vi "UI_spinWheel.vi"(8 "error in (no error)":errorcluster) -> (0 "error out":errorcluster, 2 "Cash":dbl, 3 "Spin Result":string)   [LabVIEW 2020]
uses:
  Typedefs/game_wheelItems.ctl
  <vilib>/numeric/Random Number (Range) U64.vi
  <vilib>/numeric/sub_Random U32.vi
panel:
  in  "OK":bool
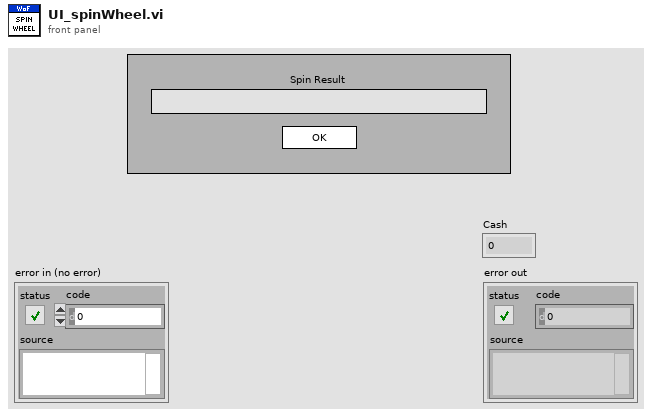
[diagram p1: front panel]
types:
  T1 = typedef "game_wheelItems.ctl" = string[]
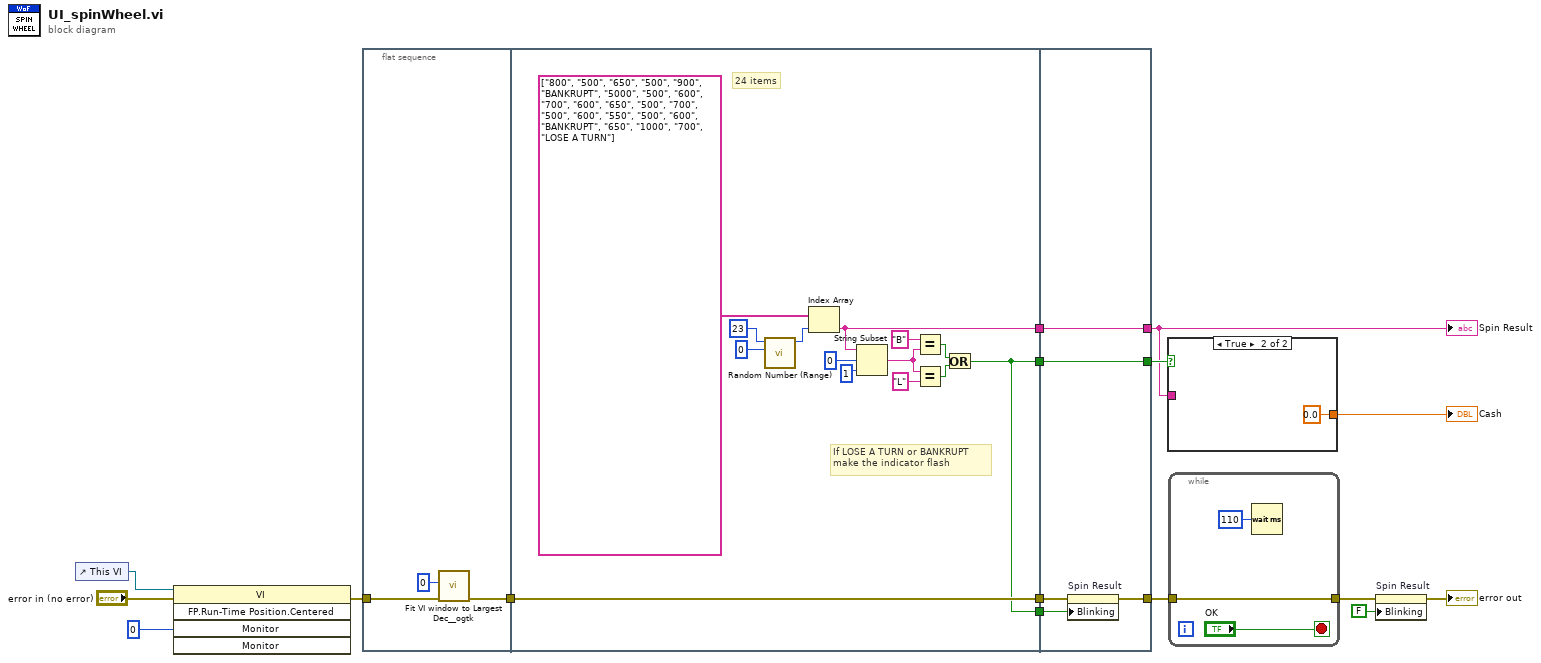
[diagram p0: block diagram]
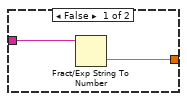
[diagram p2: hidden frame]
diagram:
  n1 = control-ref of="This VI"() -> (w1:refnum<vi>)
  n2 = invoke class="VI" method="FP.Run-Time Position.Centered"(reference=w1, error in="error in (no error)", "Monitor"=i16 0) -> (error out=w4:errorcluster)  [unwired: 2 in, 4 out]
  n3 = flat-sequence {
    tunnel: w4 -> [w18]
    tunnel: [w17] -> w16
    tunnel: w16 -> [w29]
    tunnel: [w29] -> w15
    tunnel: [w28] -> w13
    tunnel: [w20] -> w9
    tunnel: [w20] -> w8
    tunnel: w15 -> [w37]
    tunnel: [w36] -> w14
    tunnel: w13 -> [w38]
    tunnel: [w38] -> w6
    tunnel: w9 -> [w35]
    tunnel: w8 -> [w34]
    tunnel: [w34] -> w7
    frame #0 {
      n4 = call <userlib>:"Fit VI window to Largest Dec__ogtk.vi"("error in (no error)"=w18, "border spacing (2 px)"=0) -> ("error out"=w17:errorcluster)  [unwired: 4 in, 1 out]
    }
    frame #1 {
      # "If LOSE A TURN or BANKRUPT\nmake the indicator flash"
      # "24 items"
      n5 = call-poly <vilib>:"Random Number (Range).vi"("lower bound (0)"=u64 0, "upper bound (100)"=u64 23) -> ("number"=w30:u64)  [unwired: 9 in]
      n6 = Index Array(array=T1 ["800", "500", "650", "500", "900", "BANKRUPT", "5000", "500", "600", "700", "600", "650", "500", "700", "500", "600", "550", "500", "600", "BANKRUPT", "650", "1000", "700", "LOSE A TURN"] ("Array"), index=w30) -> (element=w28:string)
      n7 = String Subset(string=w28, offset (0)=0, length (rest)=1 ("length (rest)")) -> (substring=w25:string)
      n8 = Equal?(x="B", y=w25) -> (x = y?=w21:bool)
      n9 = Equal?(x=w25, y="L") -> (x = y?=w22:bool)
      n10 = Or(x=w21, y=w22) -> (x .or. y?=w20:bool)
    }
    frame #2 {
      n11 = property on="Spin Result" class="Str"(error in=w37, "Blinking"=w35) -> (error out=w36:errorcluster)  [unwired: 1 in, 1 out]
    }
  }
  n12 = case shown="True" w7 {
    tunnel: w6 -> [w40 _]
    tunnel: [w39 0.0] -> w5
    frame False {
      n13 = Fract/Exp String To Number(string=w40) -> (number=w39:dbl)  [unwired: 3 in, 1 out]
    }
    frame True {
    }
  }
  "Cash" <- w5
  n14 = while {
    tunnel: w14 -> [w42]
    tunnel: [w42] -> w12
    stop <- "OK" stop-if-true
    n15 = Wait (ms)(milliseconds to wait=u32 110) -> ()  [unwired: 1 out]
  }
  n16 = property on="Spin Result" class="Str"(error in=w12, "Blinking"=FALSE) -> (error out=→"error out":errorcluster)  [unwired: 1 in, 1 out]
  "Spin Result" <- w6
